vi "Decode Hops From TTL.vi"(0 "TTL":u8=128) -> (1 "TTL Out":u8, 2 "Hops":u8)   [LabVIEW 2018]
panel:
  # "Contains all of the functions essential to sending \n\"ping\" packets using Winsock 2 raw sockets. \n Depends on IP Checksum.vi for calculating \nIP-style checksums on blocks of data, however."
  # "Figure out how far the packet travelled"
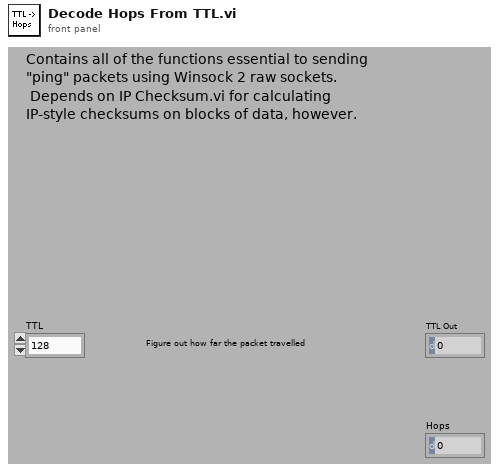
[diagram p1: front panel]
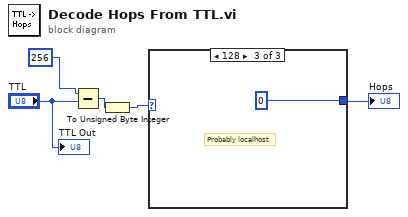
[diagram p0: block diagram]
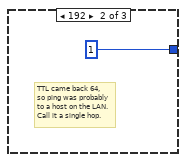
[diagram p3: hidden frame]
diagram:
  n1 = Subtract(x=u16 256, y="TTL") -> (x-y=w4:u16)
  n2 = To Unsigned Byte Integer(number=w4) -> (unsigned 8bit integer=w2:u8)
  n3 = case shown="128" w2 {
    selector: w2 -> [w6 _ _]
    tunnel: [w6 u8 1 ("x") u8 0 ("x")] -> w3
    frame 0, Default {
    }
    frame 192 {
      # "TTL came back 64, \nso ping was probably\nto a host on the LAN.\nCall it a single hop."
    }
    frame 128 {
      # "Probably localhost"
    }
  }
  "Hops" <- w3
  "TTL Out" <- "TTL"
